vi "transmit.vi"(8 "error in (no error)":errorcluster, 11 "DesktopModbus in":refnum<class "DesktopModbus.lvclass">) -> (0 "error out":errorcluster, 3 "DesktopModbus out":refnum<class "DesktopModbus.lvclass">)   [LabVIEW 2016, in "DesktopModbus.lvclass"]
uses:
  DesktopModbus.lvclass
  Common_RT_Modbus/DataTypes/TxFrame.ctl
  DesktopModbus.lvclass/DesktopModbus.ctl
  Common_RT_Modbus/DataTypes/RxFrame.ctl
  Common_RT_Modbus/RTModbus.lvlib
panel:
  out "error out 2":errorcluster
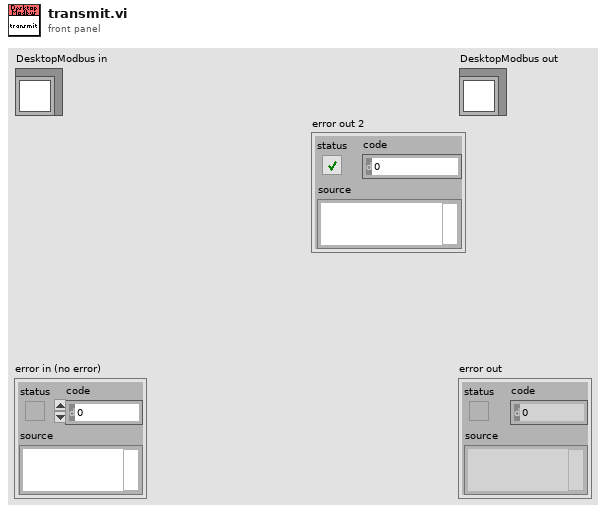
[diagram p1: front panel]
types:
  T1 = typedef "RTModbus.lvlib/TxFrame.ctl" = cluster{"Data":u8[], "WaitForTrigger":bool, "WaitForRx":u16, "TriggerIRQ":bool, "DelayMicroseconds":u16, "DelayMilliseconds":u16, "Timestamp":bool}
  T2 = typedef "RTModbus.lvlib/RxFrame.ctl" = cluster{"Data":u8[], "Timestamp":u64}
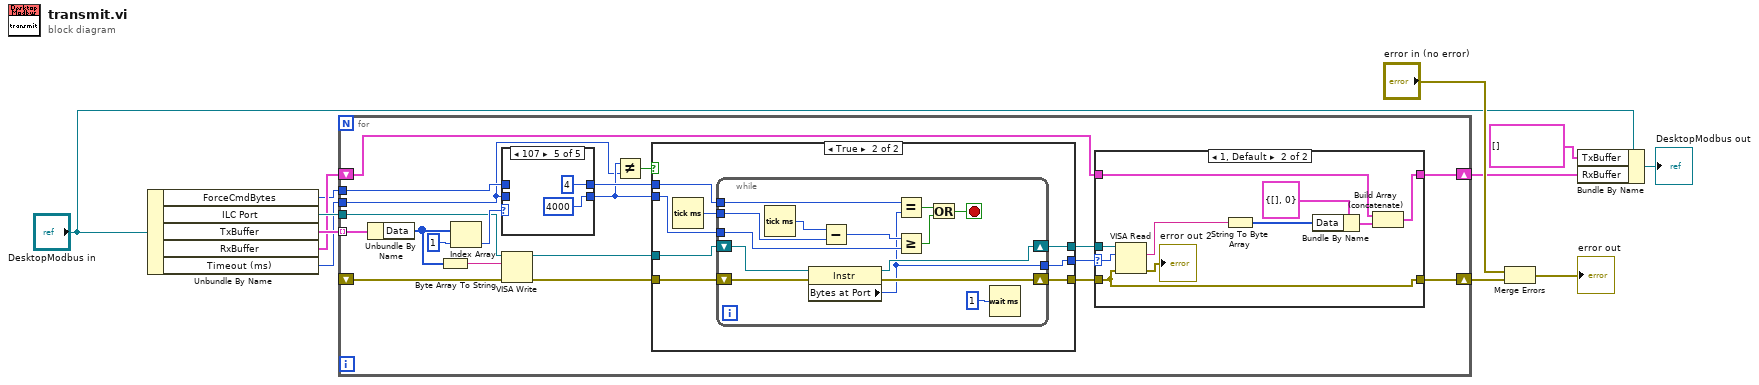
[diagram p0: block diagram]
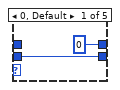
[diagram p3: hidden frame]
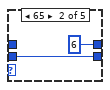
[diagram p4: hidden frame]
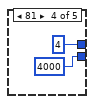
[diagram p6: hidden frame]
diagram:
  n1 = Unbundle By Name("DesktopModbus in") -> ("ForceCmdBytes"=w3:i32, "ILC Port"=w11:refnum<visa-resource-name>, "TxBuffer"=w12:T1[], "RxBuffer"=w10:T2[], "Timeout (ms)"=w2:u32)
  n2 = for {
    tunnel: w12 -> [w31] mode=indexing
    tunnel: w11 -> [w16]
    shift-right: [w29] -> w1
    shift-left: _ -> [w32]
    shift-right: [w27] -> w5
    shift-left: w10 -> [w28]
    tunnel: w3 -> [w23]
    tunnel: w2 -> [w14]
    n3 = Unbundle By Name(w31) -> ("Data"=w26:u8[])
    n4 = Byte Array To String(unsigned byte array=w26) -> (string=w30:string)
    n5 = Index Array(array=w26, index=1) -> (element=w24:u8)
    n6 = case shown="107" w24 {
      tunnel: [0 6 w63 4 ("ForceCmdBytes") 4 ("ForceCmdBytes")] -> w21
      tunnel: w23 -> [_ _ w63 _ _]
      tunnel: w14 -> [w58 w60 w62 _ _]
      tunnel: [w58 w60 w62 u32 4000 ("Timeout (ms)") u32 4000 ("Timeout (ms)")] -> w15
      frame 0, Default {
      }
      frame 65 {
      }
      frame 75 {
      }
      frame 81 {
      }
      frame 107 {
      }
    }
    n7 = VISA Write(VISA resource name=w16, write buffer=w30, error in (no error)=w32) -> (VISA resource name out=w22:refnum<visa-resource-name>, error out=w20:errorcluster)  [unwired: 1 out]
    n8 = Not Equal?(x=w15, y=w14) -> (x != y?=w13:bool)
    n9 = case shown="True" w13 {
      tunnel: w22 -> [w34 w43]
      tunnel: w21 -> [w35 w42]
      tunnel: w20 -> [w33 w41]
      tunnel: [w33 w40] -> w19
      tunnel: [w34 w39] -> w18
      tunnel: [w35 w38] -> w17
      tunnel: w15 -> [_ w37]
      frame False {
      }
      frame True {
        n10 = Tick Count (ms)() -> (millisecond timer value=w36:u32)
        n11 = while {
          tunnel: w42 -> [w56]
          shift-right: [w53] -> w39
          shift-left: w43 -> [w57]
          shift-right: [w54] -> w40
          shift-left: w41 -> [w55]
          tunnel: w36 -> [w51]
          tunnel: w37 -> [w49]
          tunnel: [w45] -> w38
          stop <- w46 stop-if-true
          n12 = Tick Count (ms)() -> (millisecond timer value=w52:u32)
          n13 = property class="Instr"(reference=w57, error in=w55) -> (reference out=w53:refnum<visa-resource-name>, error out=w54:errorcluster, "Bytes at Port"=w45:u32)
          n14 = Subtract(x=w52, y=w51) -> (x-y=w50:u32)
          n15 = Equal?(x=w56, y=w45) -> (x = y?=w48:bool)
          n16 = Greater Or Equal?(x=w50, y=w49) -> (x >= y?=w47:bool)
          n17 = Or(x=w48, y=w47) -> (x .or. y?=w46:bool)
          n18 = Wait (ms)(milliseconds to wait=u32 1) -> ()  [unwired: 1 out]
        }
      }
    }
    n19 = case shown="1, Default" w17 {
      selector: w17 -> [_ w76]
      tunnel: w19 -> [w69 w71]
      tunnel: [w69 w71] -> w29
      tunnel: w18 -> [_ w79]
      tunnel: w28 -> [w68 w78]
      tunnel: [w68 w77] -> w27
      frame 0 {
      }
      frame 1, Default {
        n20 = VISA Read(VISA resource name=w79, byte count=w76, error in (no error)=w71) -> (read buffer=w73:string, error out=→"error out 2":errorcluster)  [unwired: 2 out]
        n21 = String To Byte Array(string=w73) -> (unsigned byte array=w75:u8[])
        n22 = Bundle By Name(cluster=T2 {"Data"=[], "Timestamp"=0} ("Frame"), "Data"=w75) -> (w72:T2)
        n23 = Build Array (concatenate)(w78, w72) -> (w77:T2[])
      }
    }
  }
  n24 = Merge Errors("error in (no error)", w1) -> (→"error out":errorcluster)
  n25 = Bundle By Name(cluster="DesktopModbus in", "TxBuffer"=T1[] [], "RxBuffer"=w5) -> (→"DesktopModbus out":refnum<class "DesktopModbus.lvclass">)
